vi "K_S30_VISA F73 und F48.vi"(4 "error in":errorcluster, 6 "Channel":enum16{"CH0", "P1", "P2", "T", "TOB1", "TOB2"}(ring), 7 "Address":u8=250) -> (0 "error out":errorcluster, 1 "msg":string, 2 "Status":u8 format="%.0b", 3 "Value":sgl format="%.6e")   [LabVIEW 2012]
panel:
  # "Function 73 + F48: Read Value of a Channel\nwith automatic ini if exception 32 ocured\nV1.0, b.v."
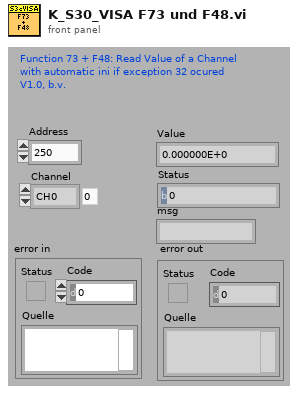
[diagram p1: front panel]
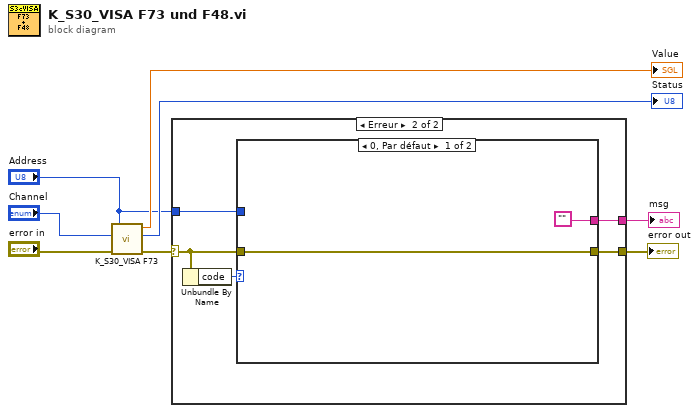
[diagram p0: block diagram]
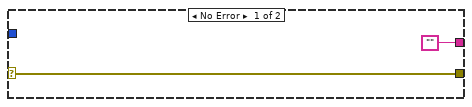
[diagram p2: hidden frame]
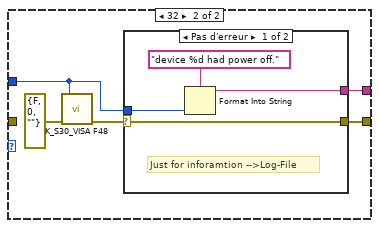
[diagram p3: hidden frame]
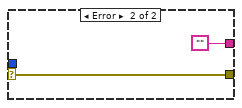
[diagram p4: hidden frame]
diagram:
  n1 = call "K_S30_VISA F73.vi"("error in"="error in", "Channel"="Channel", "Address"="Address") -> ("error out"=w3:errorcluster, "Status"=→"Status":u8, "Value"=→"Value":sgl)  [unwired: 2 in]
  n2 = case shown="Erreur" w3 {
    selector: w3 -> [w10 w13]
    tunnel: "Address" -> [_ w15]
    tunnel: [w10 w14] -> w2
    tunnel: ["" w11] -> w1
    frame No Error {
    }
    frame Error {
      n3 = Unbundle By Name(w13) -> ("code"=w12:i32)
      n4 = case shown="0, Par défaut" w12 {
        tunnel: w15 -> [_ w21]
        tunnel: w13 -> [w17 _]
        tunnel: [w17 w20] -> w14
        tunnel: ["" w18] -> w11
        frame 0, Default {
        }
        frame 32 {
          n5 = call "K_S30_VISA F48.vi"("error in"=errorcluster {"status"=FALSE, "code"=0, "source"=""}, "Address"=w21) -> ("error out"=w19:errorcluster)  [unwired: 3 in, 2 out]
          n6 = case shown="Pas d'erreur" w19 {
            selector: w19 -> [w24 w28]
            tunnel: w21 -> [w25 _]
            tunnel: [w24 w28] -> w20
            tunnel: [w23 ""] -> w18
            frame No Error {
              # "Just for inforamtion -->Log-File"
              n7 = Format Into String(format string="device %d had power off." ("Format-String"), w25) -> (resulting string=w23:string)  [unwired: 2 in, 1 out]
            }
            frame Error {
            }
          }
        }
      }
    }
  }
  "error out" <- w2
  "msg" <- w1
